vi "Stimulator Control-AO Define.vi"(4 "Sample Rate (KHz)":dbl=100.0, 5 "Amplitude (V)":dbl=5.0 format="%0.2f", 6 "Duty cycle (%)":dbl=0.03 format="%0.2f", 7 "F-STIM (Hz)":dbl=3.0 format="%0.2f", 9 "# of STIMU Train":i32=2, 10 "Interval (s)":dbl=30.0 format="%0.2f", 11 "One STIMU (s)":dbl=2.0 format="%0.2f") -> (3 "waveform out":waveform(dbl)(graph)={"t0"=timestamp(0 s since 1904-01-01), "dt"=1.0, "Y"=array[6400000 elements]})   [LabVIEW 2017]
uses:
  <vilib>/Waveform/WDTOps.llb/WDT Append Waveforms DBL.vi
  <vilib>/measure/NI_MABase.lvlib
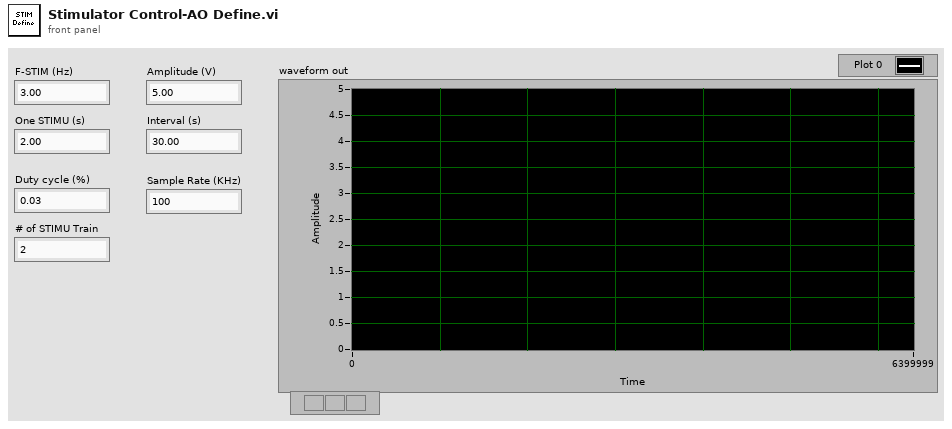
[diagram p1: front panel]
types:
  T1 = enum16{"Sine Wave", "Triangle Wave", "Square Wave", "Sawtooth Wave"}
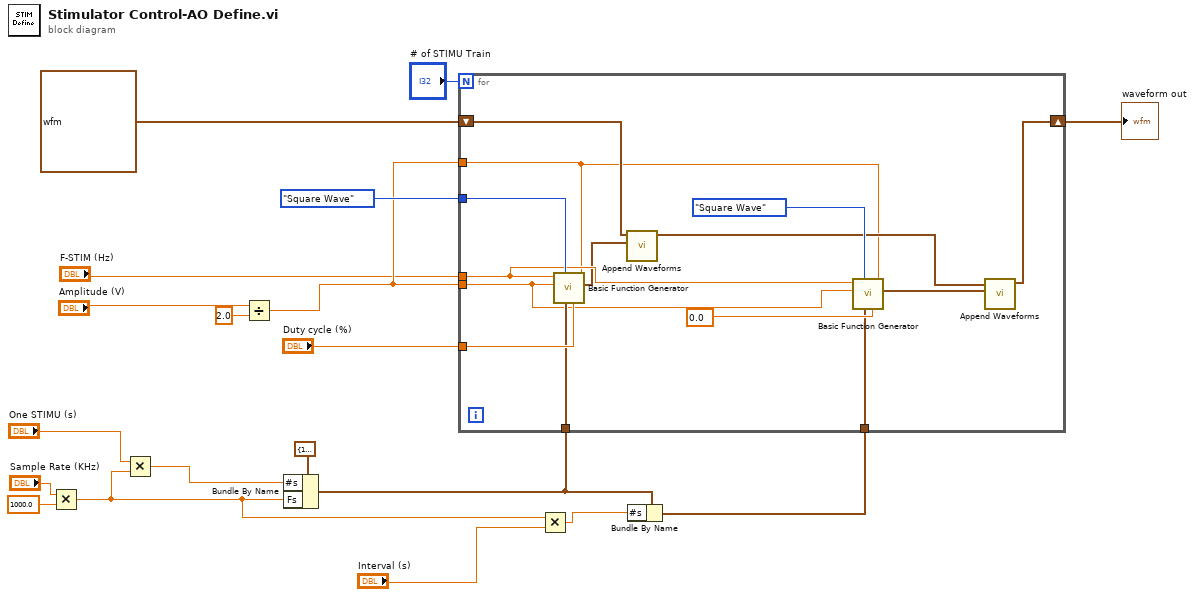
[diagram p0: block diagram]
diagram:
  n1 = Multiply(x="Sample Rate (KHz)", y=1000.0) -> (x*y=w7:dbl)
  n2 = Multiply(x="One STIMU (s)", y=w7) -> (x*y=w16:dbl)
  n3 = Divide(x="Amplitude (V)", y=2.0) -> (x/y=w6:dbl)
  n4 = Bundle By Name(cluster=cluster{"Fs":dbl, "#s":dbl} {"Fs"=1000.0, "#s"=1000.0} ("sampling info"), "#s"=w16, "Fs"=w7) -> (w13:cluster{"Fs":dbl, "#s":dbl})
  n5 = Multiply(x=w7, y="Interval (s)") -> (x*y=w11:dbl)
  n6 = Bundle By Name(cluster=w13, "#s"=w11) -> (w12:cluster{"Fs":dbl, "#s":dbl})
  n7 = for {
    N: "# of STIMU Train" -> [_]
    tunnel: w6 -> [w21]
    tunnel: T1."Square Wave" ("signal type") -> [w33]
    tunnel: "Duty cycle (%)" -> [w32]
    tunnel: w6 -> [w20]
    tunnel: w13 -> [w29]
    tunnel: w12 -> [w28]
    tunnel: "F-STIM (Hz)" -> [w27]
    shift-right: [w22] -> w8
    shift-left: waveform(dbl) {"t0"=timestamp(0 s since 1904-01-01), "dt"=1.0, "Y"=[]} ("waveform out") -> [w24]
    n8 = call <vilib>:"Basic Function Generator.vi"("offset"=w21, "square wave duty cycle (%)"=w32, "sampling info"=w29, "signal type"=w33, "amplitude"=w20, "frequency"=w27) -> ("signal out"=w25:waveform(dbl))  [unwired: 3 in, 2 out]
    n9 = call-poly <vilib>:"Append Waveforms.vi"("waveform B"=w25, "waveform A"=w24) -> ("waveform out"=w23:waveform(dbl))  [unwired: 8 in, 1 out]
    n10 = call <vilib>:"Basic Function Generator.vi"("offset"=w21, "square wave duty cycle (%)"=0.0 ("square wave duty cycle (%) 2"), "sampling info"=w28, "signal type"=T1."Square Wave", "amplitude"=w20, "frequency"=w27) -> ("signal out"=w26:waveform(dbl))  [unwired: 3 in, 2 out]
    n11 = call-poly <vilib>:"Append Waveforms.vi"("waveform B"=w26, "waveform A"=w23) -> ("waveform out"=w22:waveform(dbl))  [unwired: 8 in, 1 out]
  }
  "waveform out" <- w8
